vi "SingleFileGraphChoose.vi"(10 "Relationship":T1, 11 "XYData":cluster{"X":dbl[], "Y":dbl[]}[](array[cluster])) -> (3 "XYDataOut":cluster{"X":dbl[], "Y":dbl[]}[](array[cluster]))   [LabVIEW 2012]
doc: "单个文件中波形显示的选择，每次显示一条波形；\n\nName:蒋松\nEmail:jiangsong@outlook.com"
panel:
  out "error out":errorcluster
  in  "error in (no error)":errorcluster
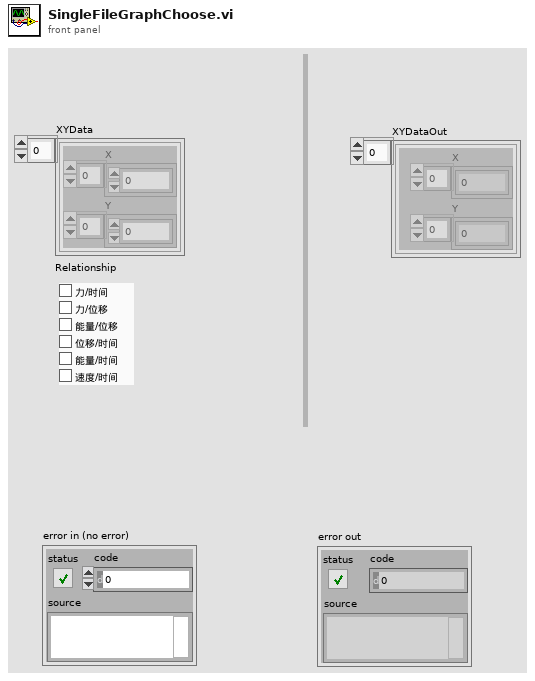
[diagram p1: front panel]
types:
  T1 = cluster{"F/T":bool, "F/D":bool, "E/D":bool, "D/T":bool, "E/T":bool, "V/T":bool}
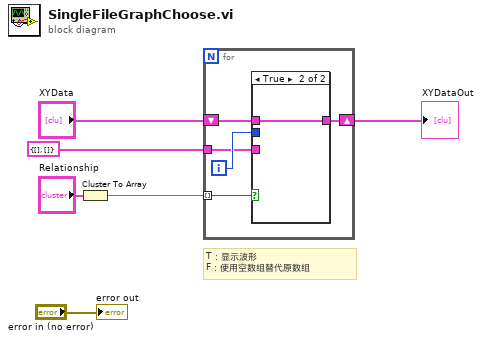
[diagram p0: block diagram]
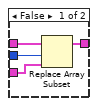
[diagram p2: hidden frame]
diagram:
  # "T：显示波形\nF：使用空数组替代原数组"
  n1 = Cluster To Array(cluster="Relationship") -> (array=w4:bool[])
  n2 = for {
    tunnel: w4 -> [w11] mode=indexing
    shift-right: [w9] -> w2
    shift-left: "XYData" -> [w10]
    tunnel: cluster{"X":dbl[], "Y":dbl[]} {"X"=[], "Y"=[]} ("new element/subarray") -> [w7]
    i -> [w8]
    n3 = case shown="True" w11 {
      tunnel: w10 -> [w15 w16]
      tunnel: [w14 w16] -> w9
      tunnel: w8 -> [w13 _]
      tunnel: w7 -> [w12 _]
      frame False {
        n4 = Replace Array Subset(array=w15, new element=w12, index=w13) -> (w14:cluster{"X":dbl[], "Y":dbl[]}[])
      }
      frame True {
      }
    }
  }
  "XYDataOut" <- w2
  "error out" <- "error in (no error)"
